vi "View.vi"(8 "error in (no error)":errorcluster, 11 "Customer In":refnum<class "Customer.lvclass">) -> (0 "error out":errorcluster)   [LabVIEW 2020, in "Customer.lvclass"]
doc: "This VI implements the main UI of the process. A reference to this VI should be set using the Set View VI Reference.vi method when the VI is started."
uses:
  Customer.lvclass
  C:/Program Files (x86)/National Instruments/LabVIEW 2020/vi.lib/Astemes/Triarc Framework/Process/Process.lvclass
  C:/Program Files (x86)/National Instruments/LabVIEW 2020/vi.lib/Astemes/Triarc Framework/View/View.lvclass
  Support/Beverages/TypeDefs/Drink Type.ctl
  Support/Beverages/TypeDefs/Options.ctl
  <vilib>/Astemes/Triarc Framework/View/View.lvclass/View.ctl
  Public/Order State.ctl
  <vilib>/Astemes/Triarc Framework/View/View.lvclass
  <vilib>/Astemes/Triarc Framework/Process/Process.lvclass
  Support/Beverages/Beverage/Beverage.lvclass
panel:
  out "All Items Received":bool
  out "Order in progress":bool
  out "Items Ordered":u32
  out "Items Received":u32
  out "Items Picked Up":string
  out "Price":dbl
  out "Order Number":u32
  in  "Reset Order":bool
  in  "Make Order":bool
  in  "Order":cluster{"Drink type":T1, "Options":T2[]}[](array[cluster])
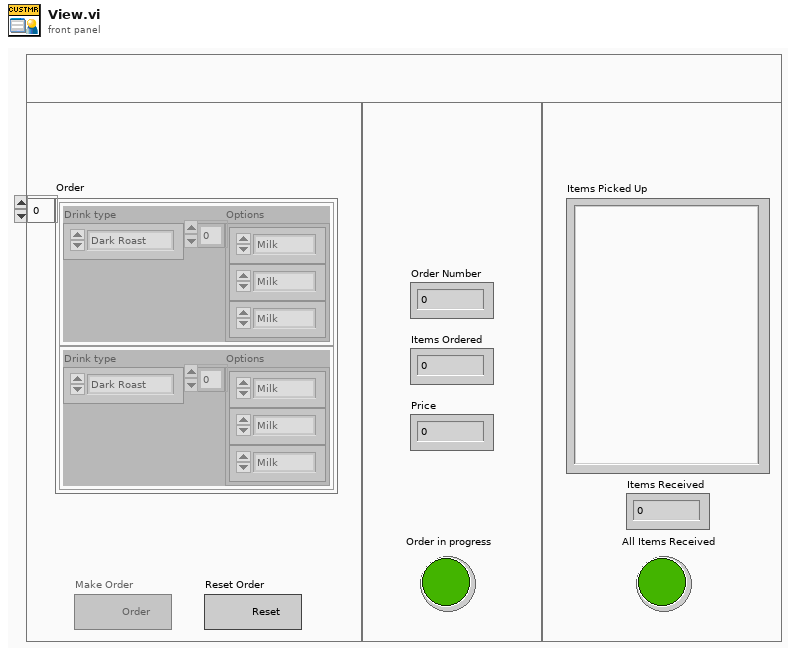
[diagram p1: front panel]
types:
  T1 = typedef "Beverage.lvclass/Drink Type.ctl" = enum16{"Dark Roast", "Decaf", "Espresso", "House Blend"}
  T2 = typedef "Beverage.lvclass/Options.ctl" = enum16{"<None>", "Milk", "Mocha", "Soy", "Whip"}
  T3 = enum8{"Enabled", "Disabled", "Disabled and Grayed Out"}
  T4 = typedef "Customer.lvclass/Order State.ctl" = cluster{"Order In Progress?":bool, "Order Number":u32, "Order Price":dbl, "Items Ordered":u32, "Items Received":u32, "Items Picked Up":string}
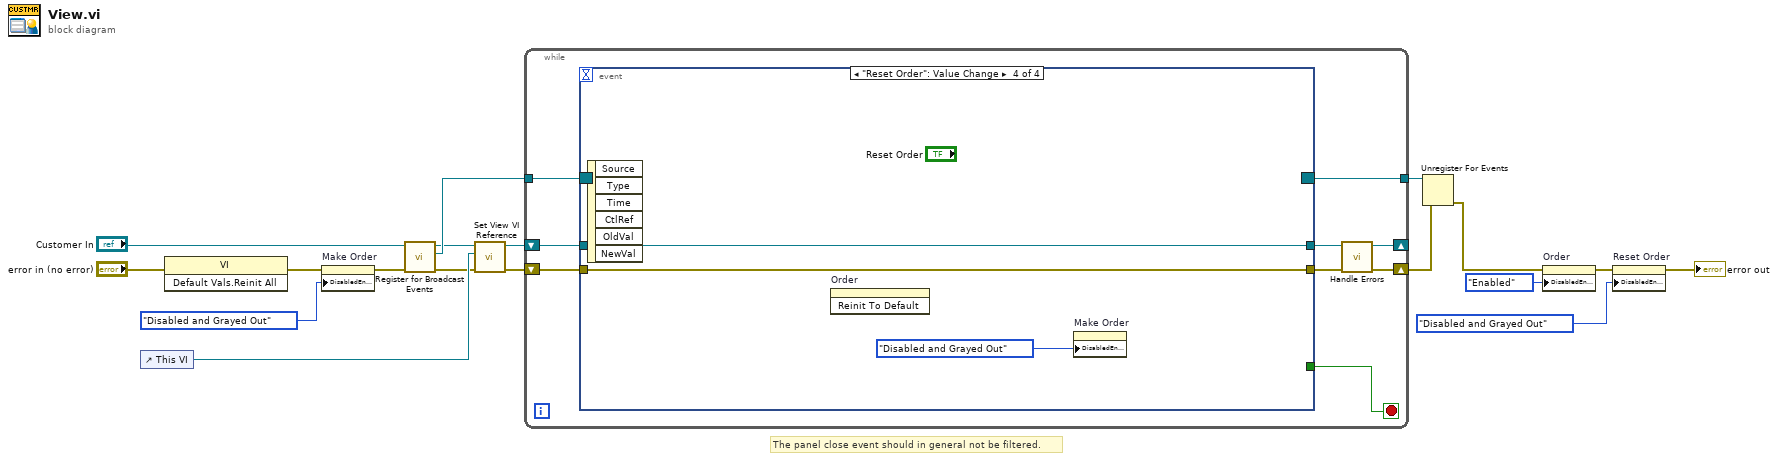
[diagram p0: block diagram]
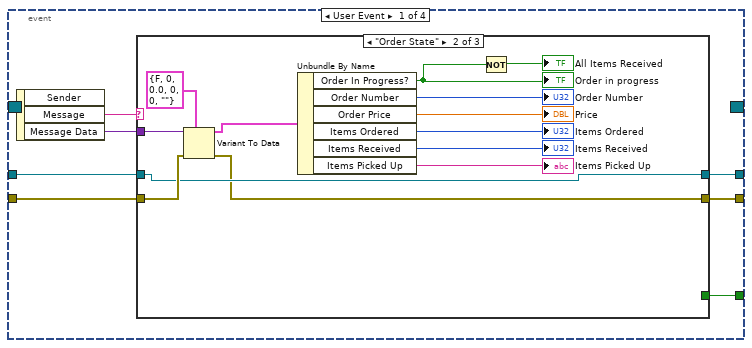
[diagram p2: hidden frame]
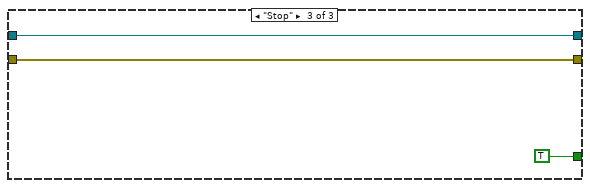
[diagram p4: hidden frame]
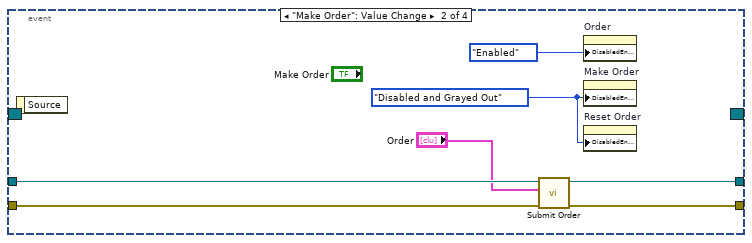
[diagram p5: hidden frame]
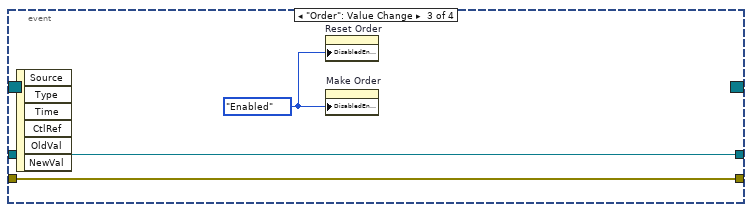
[diagram p6: hidden frame]
diagram:
  # "The panel close event should in general not be filtered."
  n1 = control-ref of="This VI"() -> (w17:refnum<vi>)
  n2 = invoke on="Invoke Node" class="VI" method="Default Vals.Reinit All"(error in="error in (no error)") -> (error out=w1:errorcluster)  [unwired: 2 in, 2 out]
  n3 = property on="Make Order" class="Bool"(error in=w1, "DisabledEnum"=T3."Disabled and Grayed Out" ("Disabled")) -> (error out=w8:errorcluster)  [unwired: 1 in, 1 out]
  n4 = call <vilib>:"Register for Broadcast Events.vi"("error in (no error)"=w8, "Process In"="Customer In") -> ("error out"=w15:errorcluster, "Event Registration Refnum Out"=w16:refnum<event-registration>, "Process Out"=w14:refnum<class "Customer.lvclass">)  [unwired: 7 in]
  n5 = call <vilib>:"Set View VI Reference.vi"("error in (no error)"=w15, "View VI Reference"=w17, "View In"=w14) -> ("error out"=w13:errorcluster, "View Out"=w12:refnum<class "Customer.lvclass">)  [unwired: 7 in]
  n6 = while {
    shift-right: [w21] -> _
    shift-left: w12 -> [w27]
    shift-right: [w19] -> w11
    shift-left: w13 -> [w25]
    tunnel: w16 -> [w24]
    tunnel: [w23] -> w10
    stop <- w22 stop-if-true
    n7 = event shown="[3] \"Reset Order\": Value Change" {
      selector: w24 -> [_ _ _ _]
      dyn-events: [_ _ _ _] -> w23
      timeout: _ -> [_ _ _ _]
      tunnel: w27 -> [w34 w56 w62 w65]
      tunnel: [w33 w57 w62 w65] -> w26
      tunnel: w25 -> [w31 w58 w61 w64]
      tunnel: [w32 w59 w61 w64] -> w20
      tunnel: [w29 _ _ _] -> w22
      event User Event {
        n8 = event-data() -> ("Message"=w30:string, "Message Data"=w28:variant)  [unwired: 1 in, 1 out]
        n9 = case shown="\"Order State\"" w30 {
          tunnel: w34 -> [w36 w39 w52]
          tunnel: [w36 w39 w52] -> w33
          tunnel: [w35 w38 w51] -> w32
          tunnel: w31 -> [w35 w48 w51]
          tunnel: [_ _ TRUE] -> w29
          tunnel: w28 -> [_ w49 _]
          frame Default {
          }
          frame "Order State" {
            n10 = Variant To Data(error in=w48, type=T4 {"Order In Progress?"=FALSE, "Order Number"=0, "Order Price"=0.0, "Items Ordered"=0, "Items Received"=0, "Items Picked Up"=""} ("Order State"), Variant=w49) -> (data=w37:T4, error out=w38:errorcluster)
            n11 = Unbundle By Name(w37) -> ("Order In Progress?"=w44:bool, "Order Number"=→"Order Number":u32, "Order Price"=→"Price":dbl, "Items Ordered"=→"Items Ordered":u32, "Items Received"=→"Items Received":u32, "Items Picked Up"=→"Items Picked Up":string)
            "Order in progress" <- w44
            n12 = Not(x=w44) -> (.not. x?=→"All Items Received":bool)
          }
          frame "Stop" {
          }
        }
      }
      event "Make Order": Value Change {
        w54 = T3."Disabled and Grayed Out" ("Disabled")
        n13 = event-data() -> ()  [unwired: 1 in, 1 out]
        n14 = call "Submit Order.vi"("error in (no error)"=w58, "Order Content"="Order", "Customer In"=w56) -> ("error out"=w59:errorcluster, "Customer Out"=w57:refnum<class "Customer.lvclass">)  [unwired: 7 in]
        n15 = property on="Order" class="Arr (strict)"("DisabledEnum"=T3."Enabled" ("Disabled")) -> ()  [unwired: 2 in, 2 out]
        n16 = property on="Make Order" class="Bool"("DisabledEnum"=w54) -> ()  [unwired: 2 in, 2 out]
        n17 = property on="Reset Order" class="Bool"("DisabledEnum"=w54) -> ()  [unwired: 2 in, 2 out]
      }
      event "Order": Value Change {
        w60 = T3."Enabled" ("Disabled")
        n18 = event-data() -> ()  [unwired: 1 in, 6 out]
        n19 = property on="Reset Order" class="Bool"("DisabledEnum"=w60) -> ()  [unwired: 2 in, 2 out]
        n20 = property on="Make Order" class="Bool"("DisabledEnum"=w60) -> ()  [unwired: 2 in, 2 out]
      }
      event "Reset Order": Value Change {
        n21 = event-data() -> ()  [unwired: 1 in, 6 out]
        n22 = invoke on="Order" class="Arr (strict)" method="Reinit To Default"() -> ()  [unwired: 3 in, 3 out]
        n23 = property on="Make Order" class="Bool"("DisabledEnum"=T3."Disabled and Grayed Out" ("Disabled")) -> ()  [unwired: 2 in, 2 out]
      }
    }
    n24 = call-dynamic "Handle Errors.vi"("error in (no error)"=w20, "Process In"=w26) -> ("error out"=w19:errorcluster, "Process Out"=w21:refnum<class "Customer.lvclass">)  [unwired: 8 in]
  }
  n25 = Unregister For Events(event registration refnum=w10, error in=w11) -> (error out=w4:errorcluster)
  n26 = property on="Order" class="Arr (strict)"(error in=w4, "DisabledEnum"=T3."Enabled" ("Disabled")) -> (error out=w5:errorcluster)  [unwired: 1 in, 1 out]
  n27 = property on="Reset Order" class="Bool"(error in=w5, "DisabledEnum"=T3."Disabled and Grayed Out" ("Disabled")) -> (error out=→"error out":errorcluster)  [unwired: 1 in, 1 out]
